vi "Actor Core.vi"(8 "error in":errorcluster, 11 "CS++StartActor in":refnum<class "CS++StartActor.lvclass">) -> (0 "error out":errorcluster, 3 "Actor out":refnum<class "Actor.lvclass">)   [LabVIEW 2013, in "CS++StartActor.lvlib" / "CS++StartActor.lvclass"]
doc: "(<B>Filename</B>: Actor Framework.lvlib:Actor.lvclass:Actor Core.vi)\n\nReceives messages to the actor, reacts to them, and initiates any error handling that may shut the actor down.\n\nDescendant classes may override this VI to append parallel tasks for the actor to complete while it handles messages. Overrides use the Call Parent Method node."
uses:
  CS++StartActor.lvclass
  <vilib>/ActorFramework/Actor/Actor.lvclass
  CS++BaseActor/CS++BaseActor.lvclass/CS++BaseActor.ctl
  CS++StartActor.lvclass/CS++StartActor.ctl
  CS++BaseActor/CS++BaseActor.lvclass
  <vilib>/ActorFramework/Actor/Actor.lvclass/Actor.ctl
  <vilib>/ActorFramework/Message Enqueuer/Message Enqueuer.lvclass/Message Enqueuer.ctl
  CS++StartActor Messages/Launch Actors Msg/Launch Actors Msg.lvclass/Launch Actors Msg.ctl
  <vilib>/ActorFramework/Message Enqueuer/Init from Existing Queue.vi
  <vilib>/ActorFramework/Message Enqueuer/Enqueue.vi
  <vilib>/ActorFramework/Message Priority Queue/Priority Enqueue.vi
  <vilib>/ActorFramework/Message Enqueuer/Message Enqueuer.lvclass
  <vilib>/ActorFramework/Stop Msg/Stop Msg.lvclass
  CS++StartActor Messages/Launch Actors Msg/Launch Actors Msg.lvclass
  CS++StartActor Messages/Launch Start Actors Msg/Launch Start Actors Msg.lvclass
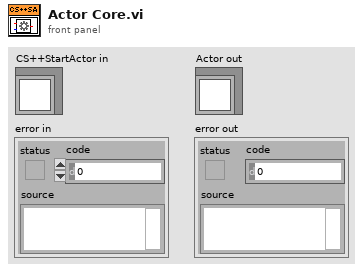
[diagram p1: front panel]
types:
  T1 = enum32{"Invalid", "Standard", "Closed", "Hidden", "Minimized", "Maximized"}
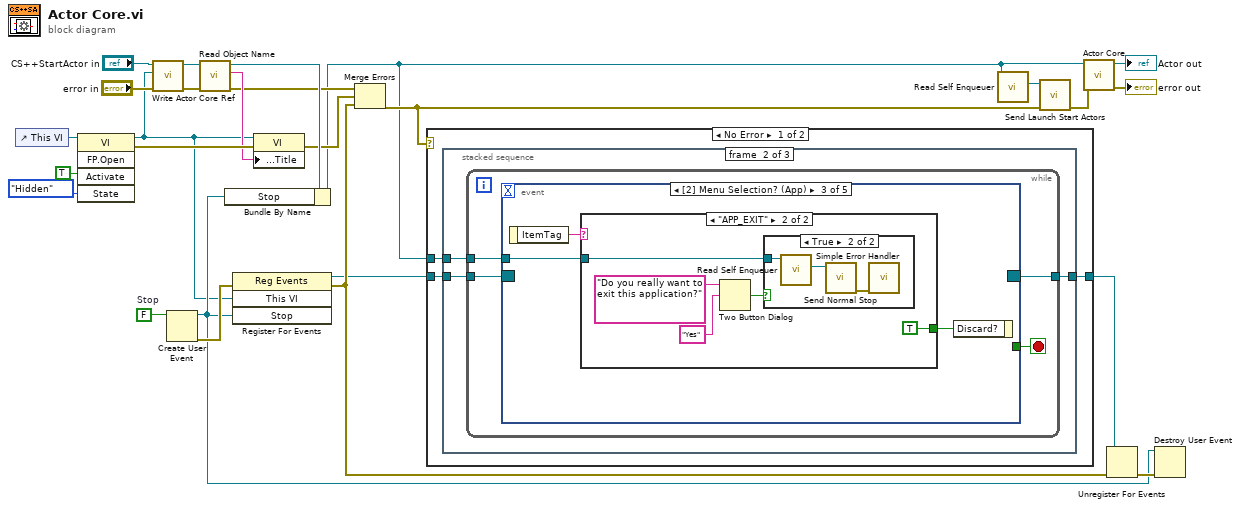
[diagram p0: block diagram]
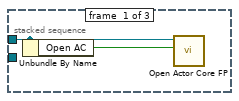
[diagram p2: hidden frame]
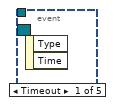
[diagram p3: hidden frame]
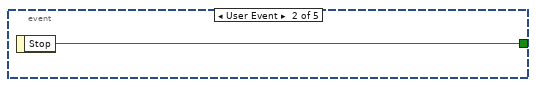
[diagram p4: hidden frame]
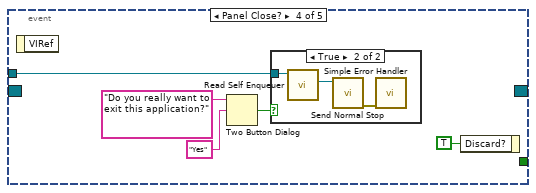
[diagram p7: hidden frame]
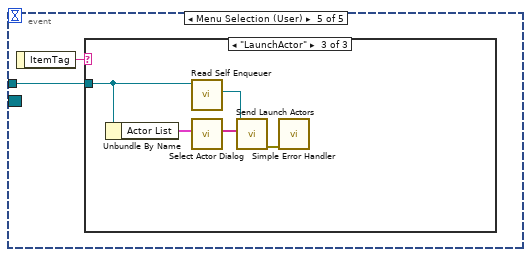
[diagram p9: hidden frame]
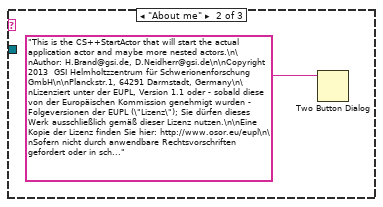
[diagram p11: hidden frame]
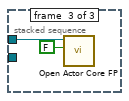
[diagram p12: hidden frame]
diagram:
  w13 = FALSE  # Stop
  n1 = control-ref of="This VI"() -> (w20:refnum<vi>)
  n2 = invoke class="VI" method="FP.Open"(reference=w20, "Activate"=TRUE ("Activate?"), "State"=T1."Hidden") -> (reference out=w1:refnum<vi>, error out=w15:errorcluster)  [unwired: 2 in, 3 out]
  n3 = call "Write Actor Core Ref.vi"("error in (no error)"="error in", "Actor Core Ref"=w1, "CS++BaseActor in"="CS++StartActor in") -> ("error out"=w17:errorcluster, "CS++BaseActor out"=w16:refnum<class "CS++StartActor.lvclass">)  [unwired: 7 in]
  n4 = Create User Event(user event datatype=w13) -> (user event=w2:refnum<user-event>, error out=w6:errorcluster)  [unwired: 1 in]
  n5 = call "Read Object Name.vi"("error in (no error)"=w17, "CS++BaseActor in"=w16) -> ("error out"=w10:errorcluster, "Object Name"=w14:string, "CS++BaseActor out"=w12:refnum<class "CS++StartActor.lvclass">)  [unwired: 7 in]
  n6 = Bundle By Name(cluster=w12, "Stop"=w2) -> (w8:refnum<class "CS++StartActor.lvclass">)
  n7 = register-events(error in=w6, w1, w2) -> (reference out=w4:refnum<event-registration>, error out=w5:errorcluster)  [unwired: 1 in]
  n8 = property class="VI"(reference=w1, error in=w15, "Front Panel.Title"=w14) -> (error out=w11:errorcluster)  [unwired: 1 out]
  n9 = Merge Errors(w10, w11, w5) -> (w9:errorcluster)
  n10 = case shown="No Error" w9 {
    tunnel: w8 -> [w29 _]
    tunnel: w4 -> [w28 w69]
    tunnel: [w27 w69] -> w3
    frame No Error {
      n11 = stacked-sequence {
        tunnel: w29 -> [w31 w33 w68]
        tunnel: w28 -> [_ w34 _]
        tunnel: [_ w32 _] -> w27
        frame #0 {
          n12 = Unbundle By Name(w31) -> ("Open AC"=w30:bool)
          n13 = call "Open Actor Core FP.vi"("Open FP (F)"=w30, "CS++BaseActor in"=w31) -> ()  [unwired: 8 in, 2 out]
        }
        frame #1 {
          n14 = while {
            tunnel: w34 -> [w38]
            tunnel: w33 -> [w37]
            tunnel: [w35] -> w32
            stop <- w36 stop-if-true
            n15 = event shown="[2] Menu Selection? (App)" {
              selector: w38 -> [_ _ _ _ _]
              dyn-events: [_ _ _ _ _] -> w35
              timeout: _ -> [_ _ _ _ _]
              tunnel: w37 -> [_ _ w42 w55 w60]
              tunnel: [_ w39 _ _ _] -> w36
              event Timeout {
                n16 = event-data() -> ()  [unwired: 1 in, 2 out]
              }
              event User Event {
                n17 = event-data() -> ("Stop"=w39:bool)  [unwired: 1 in]
              }
              event Menu Selection? (App) {
                n18 = event-data() -> ("ItemTag"=w41:string)  [unwired: 1 in]
                n19 = case shown="\"APP_EXIT\"" w41 {
                  tunnel: w42 -> [_ w47]
                  tunnel: [_ TRUE] -> w40
                  frame "False", Default {
                  }
                  frame "APP_EXIT" {
                    n20 = Two Button Dialog(message="Do you really want to exit this application?", 2:"Yes" ("T button name (\"OK\")")) -> (T button?=w46:bool)  [unwired: 1 in]
                    n21 = case shown="True" w46 {
                      tunnel: w47 -> [_ w50]
                      frame False {
                      }
                      frame True {
                        n22 = call <vilib>:"Read Self Enqueuer.vi"("Actor"=w50) -> ("Self Enqueuer"=w49:refnum<class "Message Enqueuer.lvclass">)  [unwired: 10 in]
                        n23 = call <vilib>:"Send Normal Stop.vi"("Message Enqueuer"=w49) -> ("error out"=w48:errorcluster)  [unwired: 10 in]
                        n24 = call <vilib>:"Simple Error Handler.vi"("error in (no error)"=w48) -> ()  [unwired: 4 in, 5 out]
                      }
                    }
                  }
                }
                n25 = event-data("Discard?"=w40) -> ()  [unwired: 1 in, 1 out]
              }
              event Panel Close? {
                n26 = event-data() -> ()  [unwired: 1 in, 1 out]
                n27 = Two Button Dialog(message="Do you really want to exit this application?", 2:"Yes" ("T button name (\"OK\")")) -> (T button?=w53:bool)  [unwired: 1 in]
                n28 = case shown="True" w53 {
                  tunnel: w55 -> [_ w58]
                  frame False {
                  }
                  frame True {
                    n29 = call <vilib>:"Read Self Enqueuer.vi"("Actor"=w58) -> ("Self Enqueuer"=w57:refnum<class "Message Enqueuer.lvclass">)  [unwired: 10 in]
                    n30 = call <vilib>:"Send Normal Stop.vi"("Message Enqueuer"=w57) -> ("error out"=w56:errorcluster)  [unwired: 10 in]
                    n31 = call <vilib>:"Simple Error Handler.vi"("error in (no error)"=w56) -> ()  [unwired: 4 in, 5 out]
                  }
                }
                n32 = event-data("Discard?"=TRUE) -> ()  [unwired: 1 in, 1 out]
              }
              event Menu Selection (User) {
                n33 = event-data() -> ("ItemTag"=w59:string)  [unwired: 1 in]
                n34 = case shown="\"LaunchActor\"" w59 {
                  tunnel: w60 -> [_ _ w64]
                  frame "False", Default {
                  }
                  frame "About me" {
                    n35 = Two Button Dialog(message="This is the CS++StartActor that will start the actual application actor and maybe more nested actors.\n\nAuthor: H.Brand@gsi.de, D.Neidherr@gsi.de\n\nCopyright 2013  GSI Helmholtzzentrum für Schwerionenforschung GmbH\n\nPlanckstr.1, 64291 Darmstadt, Germany\n\nLizenziert unter der EUPL, Version 1.1 oder - sobald diese von der Europäischen Kommission genehmigt wurden - Folgeversionen der EUPL (\"Lizenz\"); Sie dürfen dieses Werk ausschließlich gemäß dieser Lizenz nutzen.\n\nEine Kopie der Lizenz finden Sie hier: http://www.osor.eu/eupl\n\nSofern nicht durch anwendbare Rechtsvorschriften gefordert oder in schriftlicher Form vereinbart, wird die unter der Lizenz verbreitete Software \"so wie sie ist\", OHNE JEGLICHE GEWÄHRLEISTUNG ODER BEDINGUNGEN - ausdrücklich oder stillschweigend - verbreitet.\n\nDie sprachspezifischen Genehmigungen und Beschränkungen unter der Lizenz sind dem Lizenztext zu entnehmen.") -> ()  [unwired: 2 in, 1 out]
                  }
                  frame "LaunchActor" {
                    n36 = Unbundle By Name(w64) -> ("Actor List"=w63:cluster{"Actor Name":string, "Open":bool}[])
                    n37 = call <vilib>:"Read Self Enqueuer.vi"("Actor"=w64) -> ("Self Enqueuer"=w65:refnum<class "Message Enqueuer.lvclass">)  [unwired: 10 in]
                    n38 = call "Select Actor Dialog.vi"("Actor List"=w63) -> ("Selected Names"=w66:string[])  [unwired: 10 in]
                    n39 = call "Send Launch Actors.vi"("Selcted Actors"=w66, "Message Enqueuer"=w65) -> ("error out"=w62:errorcluster)  [unwired: 8 in, 1 out]
                    n40 = call <vilib>:"Simple Error Handler.vi"("error in (no error)"=w62) -> ()  [unwired: 4 in, 5 out]
                  }
                }
              }
            }
          }
        }
        frame #2 {
          n41 = call "Open Actor Core FP.vi"("Open FP (F)"=FALSE, "CS++BaseActor in"=w68) -> ()  [unwired: 8 in, 2 out]
        }
      }
    }
    frame Error {
    }
  }
  n42 = call <vilib>:"Read Self Enqueuer.vi"("Actor"=w8) -> ("Self Enqueuer"=w24:refnum<class "Message Enqueuer.lvclass">)  [unwired: 10 in]
  n43 = call "Send Launch Start Actors.vi"("error in (no error)"=w9, "Message Enqueuer"=w24) -> ("error out"=w23:errorcluster)  [unwired: 8 in, 1 out]
  n44 = call-parent "Actor Core.vi"("error in"=w23, "CS++BaseActor in"=w8) -> ("error out"=→"error out":errorcluster, "Actor out"=→"Actor out":refnum<class "Actor.lvclass">)  [unwired: 8 in]
  n45 = Unregister For Events(event registration refnum=w3, error in=w5) -> (error out=w7:errorcluster)
  n46 = Destroy User Event(user event=w2, error in=w7) -> ()  [unwired: 1 out]
